vi "Auto Much.vi"() -> ()   [LabVIEW 2015]
panel:
  out "Number of iteration":i32
  out "Current number":u32
  in  "Number to match":u32=50 max=1000 step=1
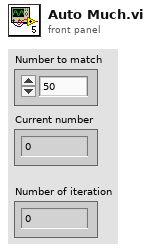
[diagram p1: front panel]
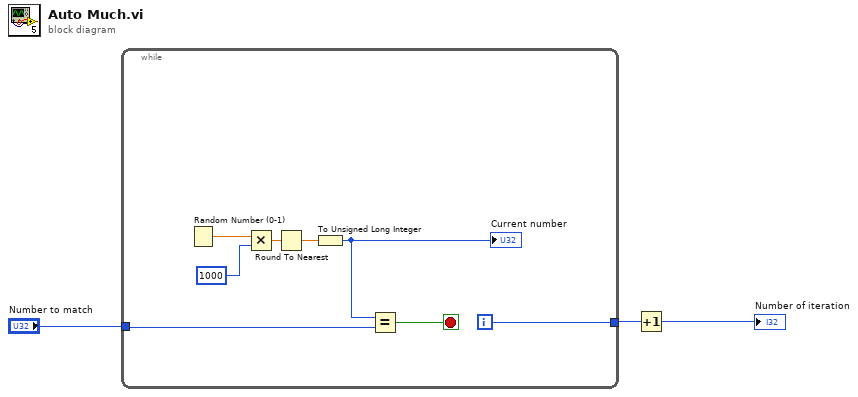
[diagram p0: block diagram]
diagram:
  n1 = while {
    tunnel: "Number to match" -> [w7]
    tunnel: [w5] -> w1
    i -> [w5]
    stop <- w6 stop-if-true
    n2 = Random Number (0-1)() -> (number: 0 to 1=w10:dbl)
    n3 = Multiply(x=w10, y=1000) -> (x*y=w9:dbl)
    n4 = Round To Nearest(number=w9) -> (nearest integer value=w8:dbl)
    n5 = To Unsigned Long Integer(number=w8) -> (unsigned 32bit integer=w4:u32)
    "Current number" <- w4
    n6 = Equal?(x=w4, y=w7) -> (x = y?=w6:bool)
  }
  n7 = Increment(x=w1) -> (x+1=→"Number of iteration":i32)
